vi "MPX.vi"() -> ()   [LabVIEW 2015]
panel:
  in  "Signal An":bool
  in  "Signalform":u16(ring)=2 items=["Sinus", "Rechteck", "SRS-Signal"]
  in  "mpX Comport":refnum<visa-resource-name>="COM5"
  in  "Amplitude [V]":i32=250
  in  "Frequenz [Hz]":i32=100
  out "read buffer":string="A200\r\nAmplitude changed\r\n\r\nWavetype: Sine\r\nFrequence: 0150 Hz\r\nAmplitude: 200,0 V\r\nSignal off\r\n\r\nempc>:\n"
  # "MPX"
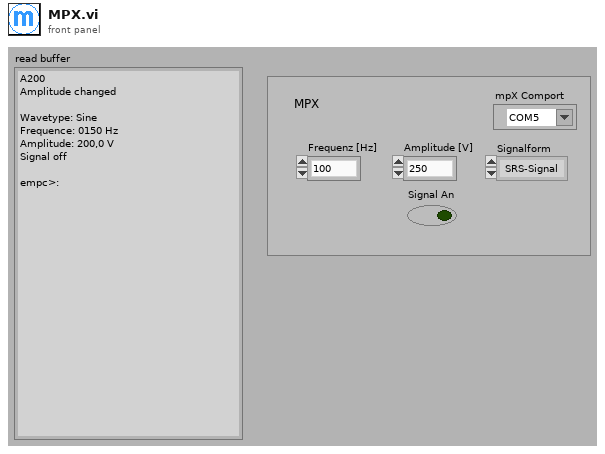
[diagram p1: front panel]
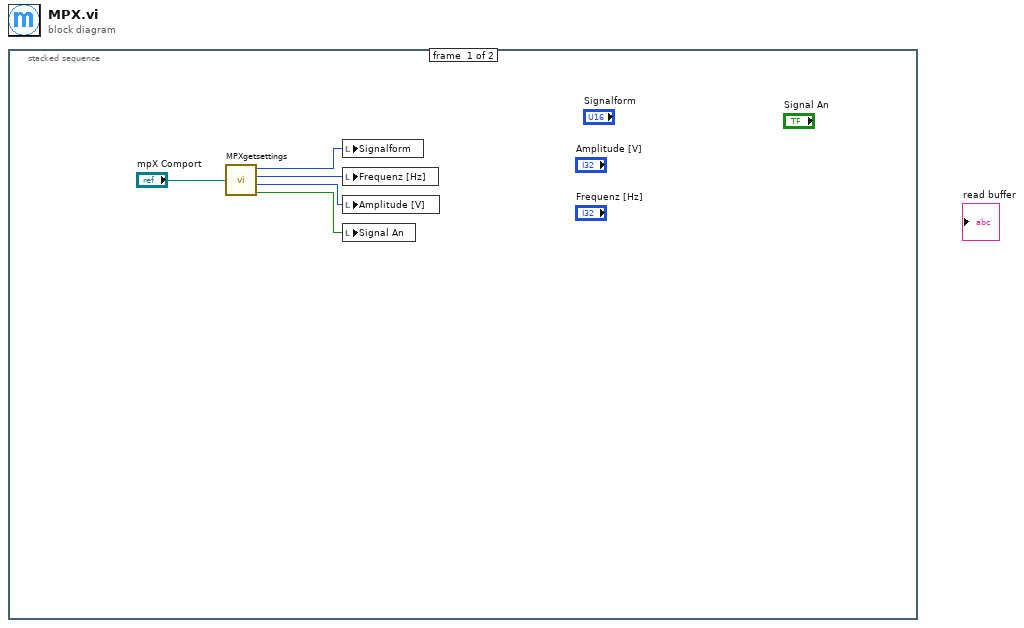
[diagram p0: block diagram]
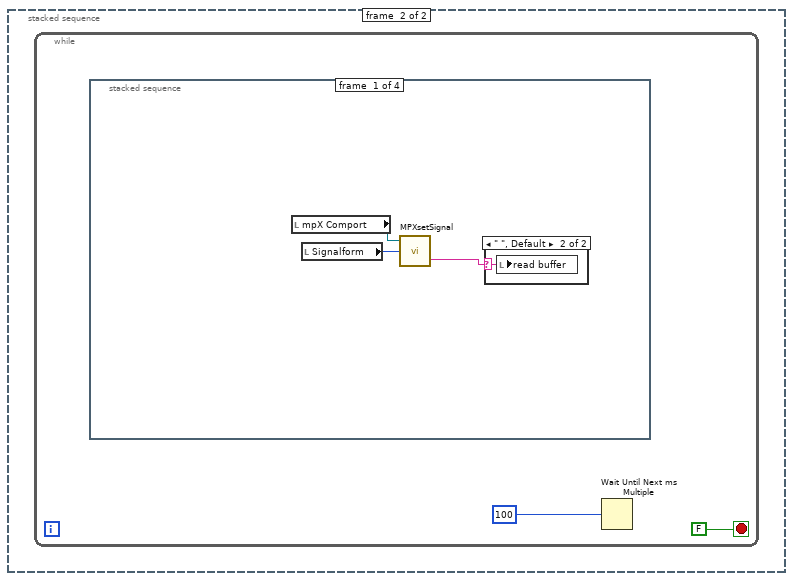
[diagram p2: hidden frame]
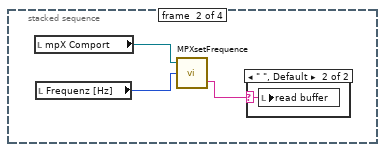
[diagram p4: hidden frame]
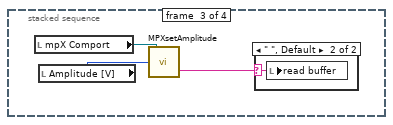
[diagram p6: hidden frame]
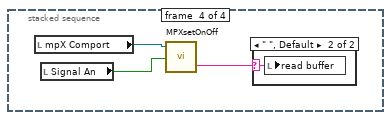
[diagram p8: hidden frame]
diagram:
  n1 = stacked-sequence {
    frame #0 {
      n2 = call "MPXgetsettings.vi"("VISA resource name"="mpX Comport") -> ("Signal On"=w2:bool, "Amplitude [V]"=w3:i32, "Frequence [Hz]"=w4:i32, "Waveform"=w5:u16)  [unwired: 1 out]
      n3 = local write "Signalform"(w5) -> ()
      n4 = local write "Frequenz [Hz]"(w4) -> ()
      n5 = local write "Amplitude [V]"(w3) -> ()
      n6 = local write "Signal An"(w2) -> ()
    }
    frame #1 {
      n7 = while {
        stop <- FALSE stop-if-true
        n8 = stacked-sequence {
          frame #0 {
            n9 = local read "mpX Comport"() -> (w9:refnum<visa-resource-name>)
            n10 = local read "Signalform"() -> (w10:u16)
            n11 = call "MPXsetSignal.vi"("Waveform"=w10, "Comport in"=w9) -> ("read buffer"=w8:string)  [unwired: 1 in, 1 out]
            n12 = case shown="\" \", Default" w8 {
              selector: w8 -> [_ w11]
              frame "" {
              }
              frame " ", Default {
                n13 = local write "read buffer"(w11) -> ()
              }
            }
          }
          frame #1 {
            n14 = local read "mpX Comport"() -> (w13:refnum<visa-resource-name>)
            n15 = local read "Frequenz [Hz]"() -> (w14:i32)
            n16 = call "MPXsetFrequence.vi"("Frequence [Hz]"=w14, "Comport in"=w13) -> ("read buffer"=w12:string)  [unwired: 1 in, 1 out]
            n17 = case shown="\" \", Default" w12 {
              selector: w12 -> [_ w15]
              frame "" {
              }
              frame " ", Default {
                n18 = local write "read buffer"(w15) -> ()
              }
            }
          }
          frame #2 {
            n19 = local read "mpX Comport"() -> (w17:refnum<visa-resource-name>)
            n20 = local read "Amplitude [V]"() -> (w18:i32)
            n21 = call "MPXsetAmplitude.vi"("Amplitude [V]"=w18, "Comport in"=w17) -> ("read buffer"=w16:string)  [unwired: 1 in, 1 out]
            n22 = case shown="\" \", Default" w16 {
              selector: w16 -> [_ w19]
              frame "" {
              }
              frame " ", Default {
                n23 = local write "read buffer"(w19) -> ()
              }
            }
          }
          frame #3 {
            n24 = local read "mpX Comport"() -> (w22:refnum<visa-resource-name>)
            n25 = local read "Signal An"() -> (w21:bool)
            n26 = call "MPXsetOnOff.vi"("Signal On"=w21, "Comport in"=w22) -> ("read buffer"=w20:string)  [unwired: 1 in, 1 out]
            n27 = case shown="\" \", Default" w20 {
              selector: w20 -> [_ w23]
              frame "" {
              }
              frame " ", Default {
                n28 = local write "read buffer"(w23) -> ()
              }
            }
          }
        }
        n29 = Wait Until Next ms Multiple(millisecond multiple=u32 100) -> ()  [unwired: 1 out]
      }
    }
  }
